vi "Global - UI Stream and Variable Connections.vi"() -> ()   [LabVIEW 2013]
uses:
  support/Message Queue/Message Cluster.ctl
  controls/Variable References.ctl
  support/Message Queue/Message Queue.lvlib
panel:
  in  "Variable References":T1 caption="变量引用"
  in  "RT Message Stream":refnum<k21> caption="RT信息流"
  in  "UI Command Stream":refnum<k21> caption="UI命令流"
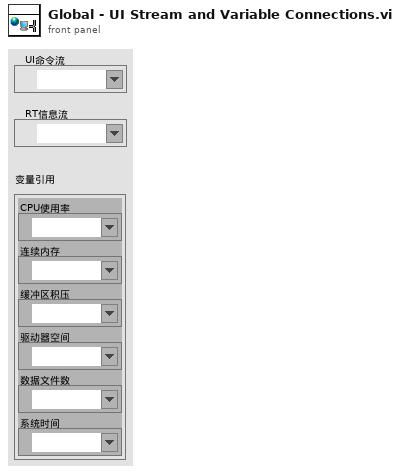
[diagram p1: front panel]
types:
  T1 = typedef "Variable References.ctl" = cluster{"CPU Usage":refnum<k21>, "Contiguous Memory":refnum<k21>, "Buffer Backlog":refnum<k21>, "Drive Space":refnum<k21>, "Number of Data Files":refnum<k21>, "System Time":refnum<k21>}
diagram:
